vi "niTuner Initialize.vi"(0 "device number":i16=1, 11 "error in":errorcluster) -> (4 "taskID out":i32 format="%.0x", 15 "error out":errorcluster {"code" format="%.0x"})   [LabVIEW 2011]
doc: "his VI initializes the PXI-5600 downconverter by loading the calibration memory, clearing the internal registers, and setting the registers to the following defaults:\n - The PXI-5600 downconverter internal clock reference is used.\n - Phase-locked loops (PLLs) are successfully locked.\n - The tuner is set to a frequency of 100 MHz with a phase detector frequency of 500 kHz.\n - Attenuation is set with a mixer level of -20 dBm and a reference level of 0 dBm.\n - The advance trigger is a software trigger.\n - The READY signal is an active low pulse of 1 ms width.\nIf all the PLLs lock correctly, the STATUS light on the PXI-5600 downconverter front panel is activated."
uses:
  nipxi5600u.dll
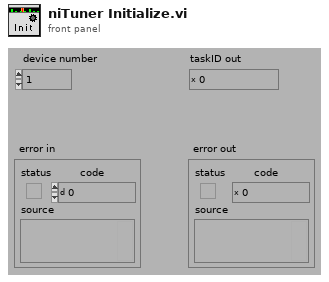
[diagram p1: front panel]
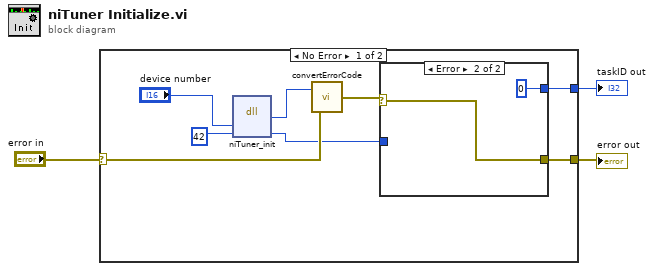
[diagram p0: block diagram]
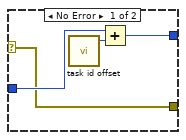
[diagram p2: hidden frame]
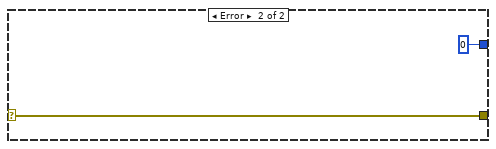
[diagram p3: hidden frame]
diagram:
  n1 = case shown="No Error" "error in" {
    selector: "error in" -> [w9 w19]
    tunnel: [w7 w19] -> w2
    tunnel: [w6 0 ("taskID")] -> w1
    frame No Error {
      n2 = dll-call lib="nipxi5600u.dll" fn="niTuner_init"("device"="device number", "taskID"=42) -> (w10:i32, "taskID"=w5:i32)  [unwired: 4 in, 2 out]
      n3 = call <instrlib>:"convertErrorCode.vi"("error in"=w9, "error code"=w10) -> ("error out"=w8:errorcluster)
      n4 = case shown="Error" w8 {
        selector: w8 -> [w12 w17]
        tunnel: [w12 w17] -> w7
        tunnel: [w14 0 ("taskID")] -> w6
        tunnel: w5 -> [w15 _]
        frame No Error {
          n5 = call <instrlib>:"task id offset.vi"() -> ("taskID offset"=w13:i32)
          n6 = Add(x=w15, y=w13) -> (x+y=w14:i32)
        }
        frame Error {
        }
      }
    }
    frame Error {
    }
  }
  "error out" <- w2
  "taskID out" <- w1
